vi "XYZStage-POSr command.vi"(7 "Number of attempts (3)":i32=3, 8 "Error in":errorcluster, 11 "VISA Refnum in":refnum<visa-resource-name>) -> (0 "Error out":errorcluster, 1 "Empty response string":bool, 2 "read string":string, 3 "VISA Refnum out":refnum<visa-resource-name>)   [LabVIEW 2020]
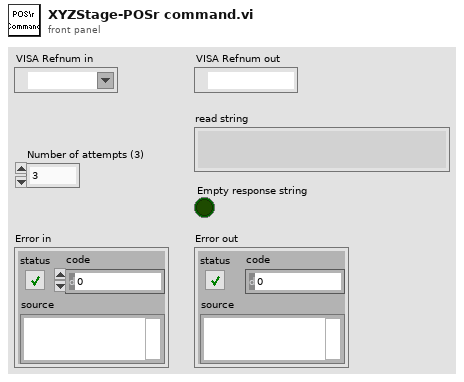
[diagram p1: front panel]
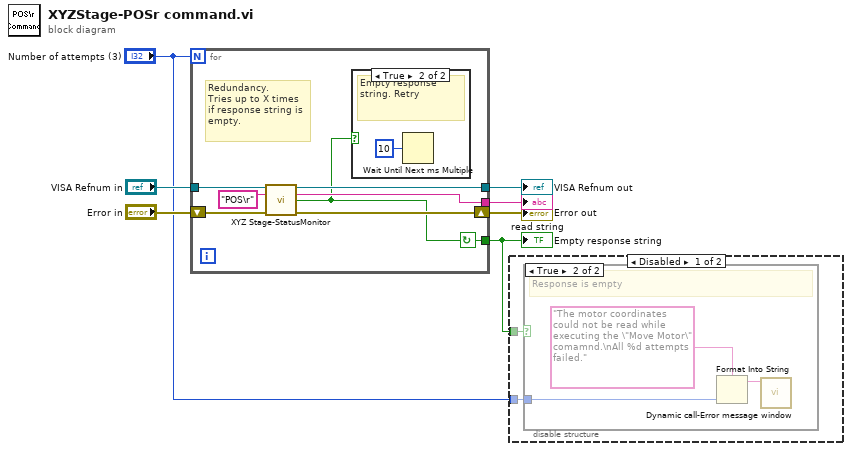
[diagram p0: block diagram]
diagram:
  n1 = for {
    N: "Number of attempts (3)" -> [_]
    tunnel: "VISA Refnum in" -> [w13]
    tunnel: [w12] -> w6
    tunnel: [w11] -> w7
    tunnel: [w8] -> w4
    shift-right: [w10] -> w3
    shift-left: "Error in" -> [w9]
    stop <- w8 continue-if-true
    # "Redundancy.\nTries up to X times\nif response string is\nempty."
    n2 = call "XYZ Stage-StatusMonitor.vi"("VISA resource name"=w13, "string to write"="POS\r", "Error In"=w9) -> ("VISA resource name out"=w11:refnum<visa-resource-name>, "read string"=w12:string, "Empty response string"=w8:bool, "Error Out"=w10:errorcluster)  [unwired: 8 in, 1 out]
    n3 = case shown="True" w8 {
      frame False {
      }
      frame True {
        # "Empty response string. Retry"
        n4 = Wait Until Next ms Multiple(millisecond multiple=u32 10) -> ()  [unwired: 1 out]
      }
    }
  }
  "Empty response string" <- w4
  "VISA Refnum out" <- w7
  "read string" <- w6
  "Error out" <- w3
  n5 = disable-structure shown="Disabled" {
    disable-tunnel: w4 -> [w17 _]
    disable-tunnel: "Number of attempts (3)" -> [w16 _]
    frame Disabled {
      n6 = case shown="True" w17 {
        tunnel: w16 -> [_ w18]
        frame False {
        }
        frame True {
          # "Response is empty"
          n7 = Format Into String(format string="The motor coordinates could not be read while executing the \"Move Motor\" comamnd.\nAll %d attempts failed." ("Error Message"), w18) -> (resulting string=w19:string)  [unwired: 2 in, 1 out]
          n8 = call "Dynamic call-Error message window.vi"("Error Message"=w19) -> ()  [unwired: 10 in, 1 out]
        }
      }
    }
    frame Enabled {
    }
  }
